vi "unpack data.vi"(10 "data":variant) -> (1 "Exposure Time (ms)":u32, 2 "cam0 Session":T1)   [LabVIEW 2020]
uses:
  <vilib>/userdefined/High Color/IMAQdx.ctl
  _controls/xiCam.ctl
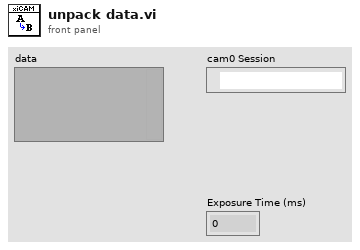
[diagram p1: front panel]
types:
  T1 = typedef "IMAQdx.ctl" = refnum<k21>
  T2 = typedef "xiCam.ctl" = cluster{"Exposure Time (ms)":u32, "cam0 Session":T1}
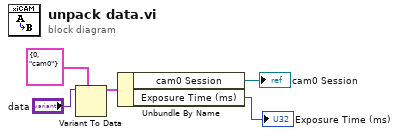
[diagram p0: block diagram]
diagram:
  n1 = Variant To Data(type=T2 {"Exposure Time (ms)"=0, "cam0 Session"="cam0"} ("Camera Controls"), Variant="data") -> (data=w2:T2)  [unwired: 1 in, 1 out]
  n2 = Unbundle By Name(w2) -> ("cam0 Session"=→"cam0 Session":T1, "Exposure Time (ms)"=→"Exposure Time (ms)":u32)
